vi "teste-motor-1.vi"() -> ()   [LabVIEW 2014]
doc: "André Romero - 2017\nandretec@ifsc.usp.br"
panel:
  out "Waveform Graph":dbl[](graph)
  out "time travel (mm/s) 2":dbl=0.04696599661844824
  out "time travel (mm/s)":dbl=0.04929751047572097
  out "time travel":u32=20285
  in  "Swap Motor":bool
  out "distance between":dbl=5.830223880587404e-05
  out "time between":u32=1007
  out "Count 2":i32=3120
  out "Count 1":i32=45033
  out "GetPOS 2":dbl=1.0 format="%_10g"
  in  "GO Move":bool
  out "IsMoving":bool
  out "GetPOS 1":dbl=1.0000583022388059 format="%_10g"
  out "Motor 2":bool
  out "Motor 1":bool
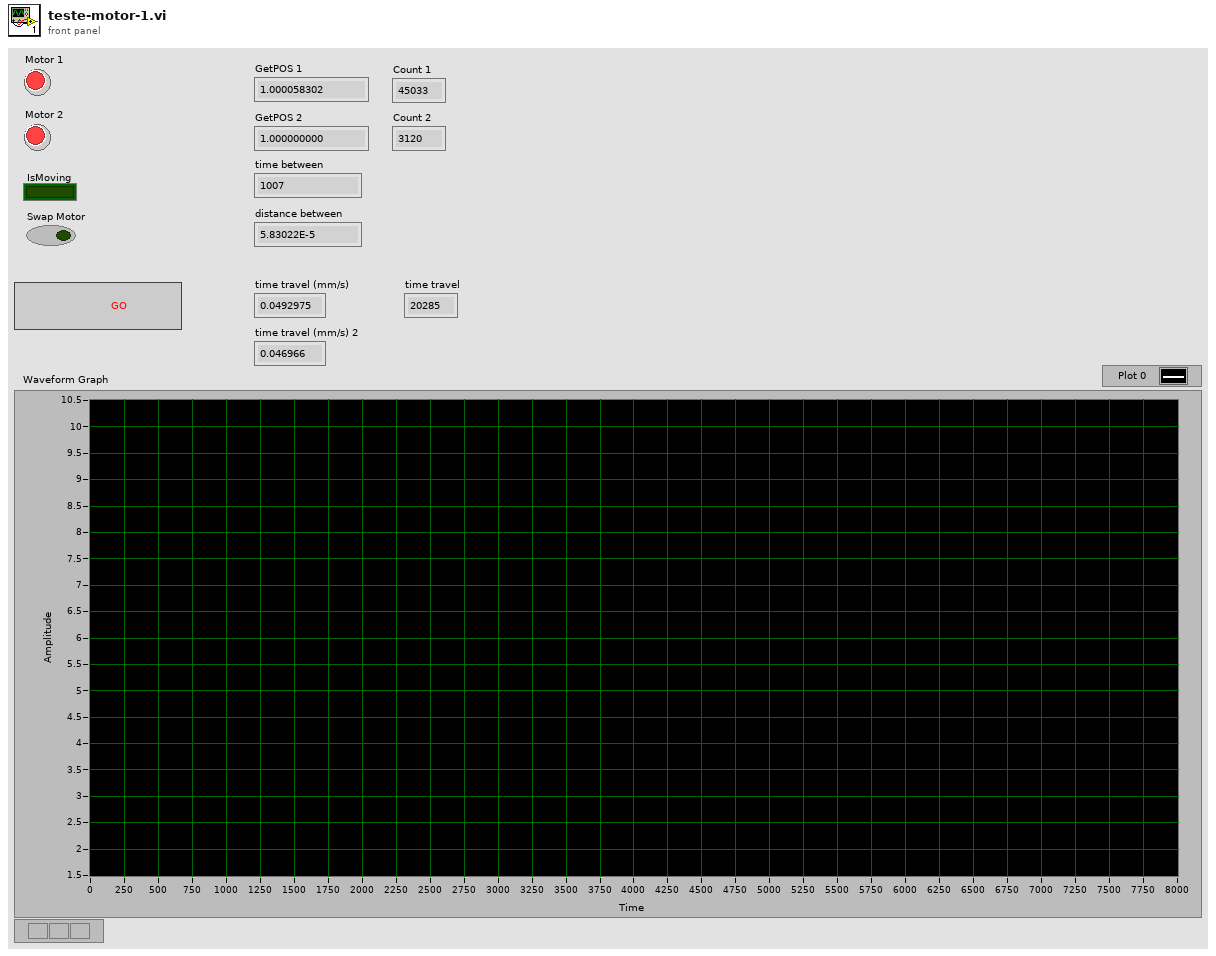
[diagram p1: front panel]
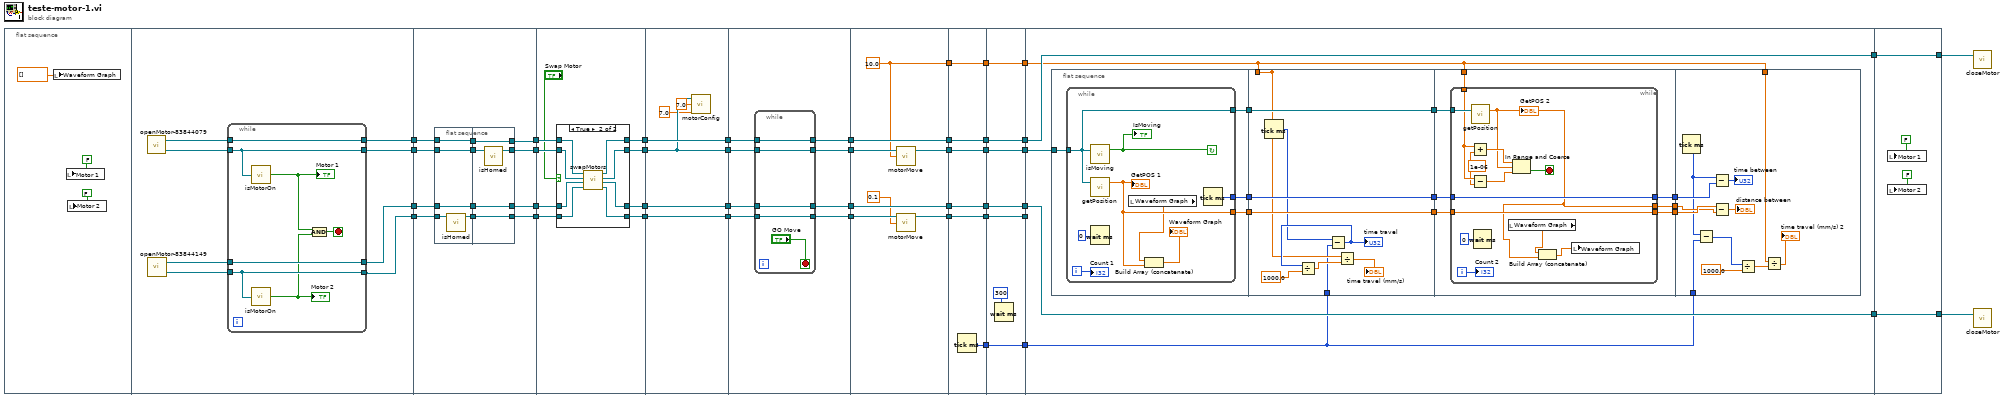
[diagram p0: block diagram]
diagram:
  n1 = flat-sequence {
    tunnel: [w50] -> w41
    tunnel: [w49] -> w40
    tunnel: [w46] -> w39
    tunnel: [w45] -> w38
    tunnel: w41 -> [w67]
    tunnel: w40 -> [w66]
    tunnel: [w69] -> w29
    tunnel: w39 -> [w68]
    tunnel: [w70] -> w28
    tunnel: w38 -> [w71]
    tunnel: [w61] -> w30
    tunnel: [w60] -> w27
    tunnel: w30 -> [w89]
    tunnel: [w90] -> w20
    tunnel: w29 -> [w85]
    tunnel: [w86] -> w18
    tunnel: w28 -> [w83]
    tunnel: [w84] -> w16
    tunnel: w27 -> [w87]
    tunnel: [w88] -> w14
    tunnel: w20 -> [w108]
    tunnel: [w108] -> w19
    tunnel: w18 -> [w107]
    tunnel: [w107] -> w17
    tunnel: w16 -> [w106]
    tunnel: [w106] -> w15
    tunnel: w14 -> [w105]
    tunnel: [w105] -> w13
    tunnel: w19 -> [w116]
    tunnel: [w115] -> w24
    tunnel: w17 -> [w112]
    tunnel: [w109] -> w23
    tunnel: w15 -> [w110]
    tunnel: [w111] -> w22
    tunnel: w13 -> [w113]
    tunnel: [w114] -> w21
    tunnel: w24 -> [w129]
    tunnel: [w129] -> w11
    tunnel: w23 -> [w128]
    tunnel: [w128] -> w9
    tunnel: w22 -> [w127]
    tunnel: [w124] -> w7
    tunnel: w21 -> [w126]
    tunnel: [w125] -> w5
    tunnel: [w122] -> w3
    tunnel: w11 -> [w135]
    tunnel: [w135] -> w10
    tunnel: w9 -> [w134]
    tunnel: [w134] -> w8
    tunnel: w7 -> [w133]
    tunnel: [w133] -> w6
    tunnel: w5 -> [w132]
    tunnel: [w132] -> w4
    tunnel: w3 -> [w131]
    tunnel: [w131] -> w2
    tunnel: [w130] -> w1
    tunnel: w10 -> [w142]
    tunnel: [w142] -> w37
    tunnel: w8 -> [w141]
    tunnel: [w141] -> w36
    tunnel: w6 -> [w140]
    tunnel: [w140] -> w35
    tunnel: w4 -> [w139]
    tunnel: [w139] -> w34
    tunnel: w2 -> [w138]
    tunnel: [w138] -> w33
    tunnel: [w136] -> w12
    tunnel: w1 -> [w136]
    tunnel: w37 -> [w152]
    tunnel: w36 -> [w151]
    tunnel: w35 -> [_]
    tunnel: w34 -> [w156]
    tunnel: w33 -> [w143]
    tunnel: [w152] -> w26
    tunnel: [w151] -> w25
    tunnel: w12 -> [w144]
    tunnel: [w213] -> w31
    tunnel: [w214] -> w32
    tunnel: w26 -> [w214]
    tunnel: w25 -> [w213]
    frame #0 {
      n2 = local write "Waveform Graph"(dbl[] [] ("Waveform Graph")) -> ()
      n3 = local write "Motor 1"(FALSE ("isConnected")) -> ()
      n4 = local write "Motor 2"(FALSE ("isConnected 2")) -> ()
    }
    frame #1 {
      n5 = call "openMotor-83844079.vi"() -> ("Device"=w51:refnum<k24>, ".NET Refnum out"=w52:refnum<k24>)  [unwired: 2 in]
      n6 = call "openMotor-83844149.vi"() -> ("Device"=w48:refnum<k24>, ".NET Refnum out"=w47:refnum<k24>)  [unwired: 2 in]
      n7 = while {
        tunnel: w52 -> [w59]
        tunnel: [w59] -> w50
        tunnel: w51 -> [w58]
        tunnel: [w58] -> w49
        tunnel: w48 -> [w56]
        tunnel: [w57] -> w46
        tunnel: w47 -> [w57]
        tunnel: [w56] -> w45
        stop <- w53 stop-if-true
        n8 = call "isMotorOn.vi"("Device"=w58) -> ("isConnected"=w54:bool)
        "Motor 1" <- w54
        n9 = call "isMotorOn.vi"("Device"=w56) -> ("isConnected"=w55:bool)
        "Motor 2" <- w55
        n10 = And(x=w54, y=w55) -> (x .and. y?=w53:bool)
      }
    }
    frame #2 {
      n11 = flat-sequence {
        tunnel: w71 -> [w76]
        tunnel: w68 -> [w74]
        tunnel: w67 -> [w73]
        tunnel: w66 -> [w72]
        tunnel: [w75] -> w65
        tunnel: [w74] -> w64
        tunnel: [w73] -> w63
        tunnel: [w72] -> w62
        tunnel: [w77] -> w60
        tunnel: [w79] -> w61
        tunnel: [w80] -> w69
        tunnel: [w81] -> w70
        tunnel: w65 -> [w81]
        tunnel: w64 -> [w80]
        tunnel: w63 -> [w79]
        tunnel: w62 -> [w78]
        frame #0 {
          n12 = call "isHomed.vi"("Device in"=w76) -> ("Device out"=w75:refnum<k24>)  [unwired: 4 in]
        }
        frame #1 {
          n13 = call "isHomed.vi"("Device in"=w78) -> ("Device out"=w77:refnum<k24>)  [unwired: 4 in]
        }
      }
    }
    frame #3 {
      n14 = case shown="True" "Swap Motor" {
        tunnel: [w94 w98] -> w90
        tunnel: w89 -> [w94 w102]
        tunnel: [w93 w97] -> w88
        tunnel: w87 -> [w93 w101]
        tunnel: [w92 w95] -> w86
        tunnel: w85 -> [w92 w100]
        tunnel: [w91 w96] -> w84
        tunnel: w83 -> [w91 w99]
        frame False {
        }
        frame True {
          n15 = call "swapMotors.vi"("Device 2"=w99, ".NET Refnum in 2"=w100, "Device 1"=w101, ".NET Refnum in 1"=w102) -> ("Device out 1"=w96:refnum<k24>, ".NET Refnum out 1"=w95:refnum<k24>, "Device out 2"=w97:refnum<k24>, ".NET Refnum out 2"=w98:refnum<k24>)
        }
      }
    }
    frame #4 {
      n16 = call "motorConfig.vi"("Velocity"=7.0 ("MaxVelocity"), "Acceleration"=7.0, "Device in"=w105) -> ()  [unwired: 2 in, 1 out]
    }
    frame #5 {
      n17 = while {
        tunnel: [w120] -> w115
        tunnel: w116 -> [w120]
        tunnel: [w119] -> w114
        tunnel: w113 -> [w119]
        tunnel: w112 -> [w117]
        tunnel: [w118] -> w111
        tunnel: w110 -> [w118]
        tunnel: [w117] -> w109
        stop <- "GO Move" stop-if-true
      }
    }
    frame #6 {
      w122 = 10.0 ("position")
      n18 = call "motorMove.vi"("position"=w122, "Device in"=w126) -> ("Device out"=w125:refnum<k24>)  [unwired: 3 in]
      n19 = call "motorMove.vi"("position"=0.1, "Device in"=w127) -> ("Device out"=w124:refnum<k24>)  [unwired: 3 in]
    }
    frame #7 {
      n20 = Tick Count (ms)() -> (millisecond timer value=w130:u32)
    }
    frame #8 {
      n21 = Wait (ms)(milliseconds to wait=u32 300) -> ()  [unwired: 1 out]
    }
    frame #9 {
      n22 = flat-sequence {
        tunnel: w156 -> [w160]
        tunnel: [w159] -> w150
        tunnel: [w158] -> w148
        tunnel: [w157] -> w146
        tunnel: w150 -> [w178]
        tunnel: [w178] -> w149
        tunnel: w148 -> [w177]
        tunnel: [w177] -> w147
        tunnel: w146 -> [w176]
        tunnel: [w176] -> w145
        tunnel: [w171] -> _
        tunnel: w143 -> [w171]
        tunnel: w144 -> [w169]
        tunnel: w149 -> [w185]
        tunnel: [w184] -> w155
        tunnel: w147 -> [w183]
        tunnel: w143 -> [w182]
        tunnel: w145 -> [w181]
        tunnel: [w180] -> w154
        tunnel: [w179] -> w153
        tunnel: w155 -> [w210]
        tunnel: w154 -> [w208]
        tunnel: w153 -> [w207]
        tunnel: w144 -> [w204]
        tunnel: w143 -> [w200]
        frame #0 {
          n23 = while {
            tunnel: w160 -> [w166]
            tunnel: [w166] -> w159
            tunnel: [w164] -> w158
            tunnel: [w163] -> w157
            i -> [w165]
            stop <- w168 continue-if-true
            n24 = call "isMoving.vi"("Device in"=w166) -> ("IsMoving"=w168:bool)  [unwired: 2 in]
            "IsMoving" <- w168
            n25 = call "getPosition.vi"("Device"=w166) -> ("GetPOS"=w163:dbl)  [unwired: 2 in]
            "GetPOS 1" <- w163
            n26 = Wait (ms)(milliseconds to wait=u32 0) -> ()  [unwired: 1 out]
            n27 = local read "Waveform Graph"() -> (w161:dbl[])
            n28 = Build Array (concatenate)(w161, w163) -> (→"Waveform Graph":dbl[])
            n29 = Tick Count (ms)() -> (millisecond timer value=w164:u32)
            "Count 1" <- w165
          }
        }
        frame #1 {
          n30 = Tick Count (ms)() -> (millisecond timer value=w170:u32)
          n31 = Subtract(x=w170, y=w169) -> (x-y=w174:u32)
          "time travel" <- w174
          n32 = Divide(x=w174, y=1000.0) -> (x/y=w175:dbl)
          n33 = Divide(x=w171, y=w175) -> (x/y=→"time travel (mm/s)":dbl)
        }
        frame #2 {
          n34 = while {
            tunnel: w185 -> [w198]
            tunnel: [w193] -> w184
            tunnel: w183 -> [w193]
            tunnel: w182 -> [w192]
            tunnel: w181 -> [w195]
            tunnel: [w195] -> w180
            tunnel: [w187] -> w179
            i -> [w197]
            stop <- w189 stop-if-true
            w191 = 1e-06
            n35 = call "getPosition.vi"("Device"=w198) -> ("GetPOS"=w187:dbl)  [unwired: 2 in]
            "GetPOS 2" <- w187
            n36 = Add(x=w192, y=w191) -> (x+y=w194:dbl)
            n37 = Subtract(x=w192, y=w191) -> (x-y=w190:dbl)
            n38 = Wait (ms)(milliseconds to wait=u32 0) -> ()  [unwired: 1 out]
            n39 = local read "Waveform Graph"() -> (w188:dbl[])
            n40 = In Range and Coerce(upper limit=w194, x=w187, lower limit=w190) -> (In Range?=w189:bool)  [unwired: 1 out]
            n41 = Build Array (concatenate)(w188, w187) -> (w186:dbl[])
            n42 = local write "Waveform Graph"(w186) -> ()
            "Count 2" <- w197
          }
        }
        frame #3 {
          n43 = Tick Count (ms)() -> (millisecond timer value=w205:u32)
          n44 = Subtract(x=w205, y=w204) -> (x-y=w202:u32)
          n45 = Subtract(x=w205, y=w210) -> (x-y=→"time between":u32)
          n46 = Subtract(x=w208, y=w207) -> (x-y=→"distance between":dbl)
          n47 = Divide(x=w202, y=1000.0) -> (x/y=w201:dbl)
          n48 = Divide(x=w200, y=w201) -> (x/y=→"time travel (mm/s) 2":dbl)
        }
      }
    }
    frame #10 {
      n49 = local write "Motor 1"(FALSE ("Motor 1 On")) -> ()
      n50 = local write "Motor 2"(FALSE ("Motor 2 On")) -> ()
    }
  }
  n51 = call "closeMotor.vi"(".NET Refnum in"=w32) -> ()  [unwired: 2 in]
  n52 = call "closeMotor.vi"(".NET Refnum in"=w31) -> ()  [unwired: 2 in]
